vi "uSubscription Update.vi"(8 "error in (no error)":errorcluster, 10 "uMsg":refnum<class "uMsg.lvclass">, 11 "uSubscription in":refnum<class "uSubscription.lvclass">) -> (0 "error out":errorcluster)   [LabVIEW 2023, in "uLib.lvlib" / "uSubscription.lvclass"]
doc: "Translates the message and sends it out."
uses:
  uSubscription.lvclass
  uMsg/uMsg/uMsg.lvclass
  uSubscription.lvclass/uSubscription.ctl
  uMsg/uMsg/uMsg.lvclass/uMsg.ctl
  uNotifyMode/uNotifyMode/uNotifyMode.lvclass/uNotifyMode.ctl
  uTransport/uTransport_uActor/uTransport_uActor.lvclass/uTransport_uActor.ctl
  uTransport/uTransport_Event/uTransport_Event.lvclass/uTransport_Event.ctl
  uTransport/uTransport_Queue/uTransport_Queue.lvclass/uTransport_Queue.ctl
  uTransport/uTransport/uTransport_SendMsg.vi
  uTransport/uTransport_uActor/uTransport_uActor_SendMsg.vi
  uTransport/uTransport_Event/uTransport_Event_SendMsg.vi
  uTransport/uTransport_Queue/uTransport_Queue_SendMsg.vi
  uMsg/uMsg/uMsg Update Timestamp.vi
  uTransport/uTransport_uActor/uTransport_uActor.lvclass
  uTransport/uTransport_Event/uTransport_Event.lvclass
  uTransport/uTransport_Queue/uTransport_Queue.lvclass
  uNotifyMode/uNotifyMode/uNotifyMode.lvclass
  uTransport/uTransport/uTransport.lvclass
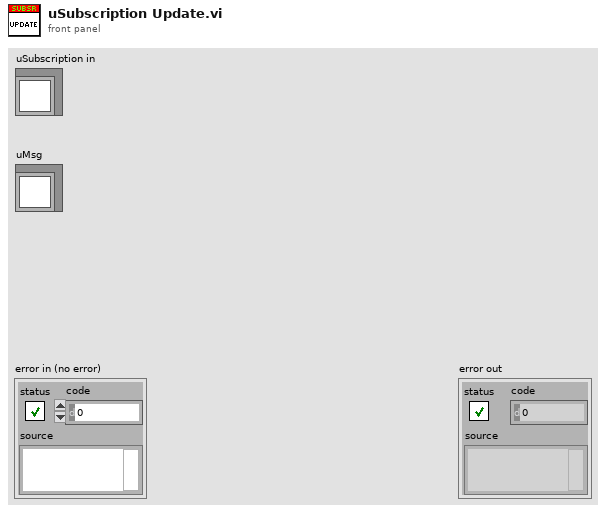
[diagram p1: front panel]
types:
  T1 = typedef "uLib.lvlib/uSubscription.lvclass/TypeDef_uSubscriptionPrivateData.ctl" = cluster{"Destination CMD":string, "uNotifyMode":refnum<class "uNotifyMode.lvclass">, "Destination uTransport":refnum<class "uTransport.lvclass">}
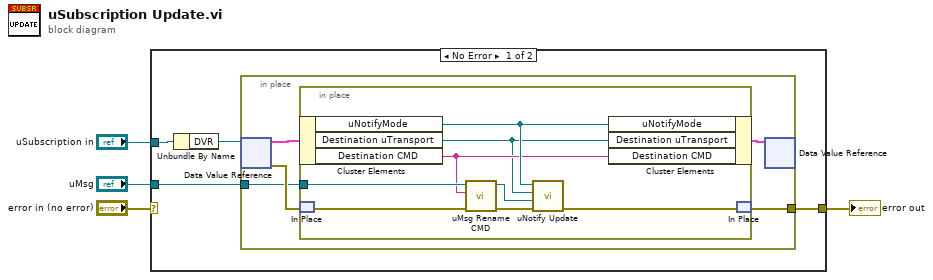
[diagram p0: block diagram]
diagram:
  n1 = case shown="No Error" "error in (no error)" {
    selector: "error in (no error)" -> [_ w22]
    tunnel: [w8 w22] -> w3
    tunnel: "uSubscription in" -> [w7 _]
    tunnel: "uMsg" -> [w6 _]
    frame No Error {
      n2 = Unbundle By Name(w7) -> ("DVR"=w5:refnum<data-value>)
      n3 = in-place {
        in-place-border: [w11] -> w8
        in-place-border: w6 -> [w9]
        n4 = in-place-dvr #1(w5) -> (w13:T1, w12:errorcluster)
        n5 = in-place {
          in-place-border: w9 -> [w16]
          n6 = in-place-cluster #2(w13) -> ("uNotifyMode"=w17:refnum<class "uNotifyMode.lvclass">, "Destination uTransport"=w14:refnum<class "uTransport.lvclass">, "Destination CMD"=w15:string)
          n7 = in-place-match #3(w12) -> (w19:errorcluster)
          n8 = call "uMsg Rename CMD.vi"("error in (no error)"=w19, "New CMD"=w15, "uMsg in"=w16) -> ("error out"=w21:errorcluster, "uMsg out"=w20:refnum<class "uMsg.lvclass">)  [unwired: 7 in]
          n9 = call "uNotify Update.vi"("error in (no error)"=w21, "Destination uMsg"=w20, "uTransport in"=w14, "uNotifyMode in"=w17) -> ("error out"=w18:errorcluster)  [unwired: 7 in]
          n10 = in-place-cluster #2("uNotifyMode"=w17, "Destination uTransport"=w14, "Destination CMD"=w15) -> (w10:T1)
          n11 = in-place-match #3(w18) -> (w11:errorcluster)
        }
        n12 = in-place-dvr #1(w10) -> ()  [unwired: 2 out]
      }
    }
    frame Error {
    }
  }
  "error out" <- w3
